vi "PXI_Host_Cluster_40_I8_Read_NewMethod_Benchmark.vi"() -> ()   [LabVIEW 2018]
uses:
  <vilib>/Platform/TimedLoop/XDataNode/timing_clust.ctl
  <vilib>/Platform/TimedLoop/XDataNode/nitl_modes.ctl
  <vilib>/Platform/TimedLoop/XDataNode/wakeup.ctl
  cRIO RT/TypeDefs/Big I8 Cluster.ctl
  acadbf34-ec47-4be6-aee9-0dde4c7960f7.vi
  cRIO RT/FPGA Bitfile Register Operations/Scalar IO Operations/SubVIs/Convert Cluster BLOB to Bool Array.vi
  cRIO RT/FPGA Bitfile Register Operations/Scalar IO Operations/SubVIs/Parse Cluster Configuration.vi
  cRIO RT/FPGA Bitfile Register Operations/Scalar IO Operations/Read Methods/Read Data Register/Instances/Read U8 Array.vi
  acadbf34-ec47-4be6-aee9-0dde4c7960f7.vi/8df46875-ca50-46a7-81d4-ea56393d8c37.vi
  cRIO RT/FPGA Bitfile Register Operations/Scalar IO Operations/SubVIs/Check Cluster Configuration Store.vi
  cRIO RT/FPGA Bitfile Register Operations/Scalar IO Operations/Utilities/Find Register Offset.vi
  cRIO RT/FPGA Bitfile Register Operations/Scalar IO Operations/SubVIs/FXP Raw to DBL.vi
  cRIO RT/FPGA Bitfile Register Operations/Scalar IO Operations/SubVIs/Check Register Data Store.vi
  <userlib>/_OpenG.lib/lvdata/lvdata.llb/Variant to Header Info__ogtk.vi
  <userlib>/_OpenG.lib/lvdata/lvdata.llb/Split Cluster TD__ogtk.vi
  <userlib>/_OpenG.lib/lvdata/lvdata.llb/Cluster to Array of VData__ogtk.vi
  <vilib>/Utility/Data Type/Get Type Information.vi
  <userlib>/_OpenG.lib/lvdata/lvdata.llb/Get Strings from Enum__ogtk.vi
  cRIO RT/FPGA Bitfile Register Operations/Scalar IO Operations/Error Handling/Error 6004.vi
  <vilib>/Utility/Data Type/Get Fixed-Point Information.vi
  cRIO RT/FPGA Bitfile Register Operations/Scalar IO Operations/Error Handling/Error 6001.vi
  cRIO RT/FPGA Bitfile Register Operations/Scalar IO Operations/Error Handling/Error 6000.vi
  cRIO RT/FPGA Bitfile Register Operations/Scalar IO Operations/Error Handling/Error 6002.vi
  cRIO RT/FPGA Bitfile Register Operations/Scalar IO Operations/Error Handling/Error 6003.vi
  <vilib>/FPGAPlugInAG/Dynamic/niLvFpga_Close_Dynamic.vi
  <vilib>/platform/TimedLoop/XDataNode/XDataNode.xnode
  <vilib>/rvi/interface/nirviCloseFPGA/nirviCloseFPGA.xnode
  cRIO RT/FPGA Bitfile Register Operations/Scalar IO Operations/FPGA Register IO.lvlib
  <vilib>/Platform/TimedLoop/XDataNode/XDNodeRunTimeDep.lvlib
panel:
  out "Waveform Graph":dbl[](graph)
  out "Standard Dev":dbl
  out "Execution time (s)":dbl
  out "Maximum(s)":dbl
  out "error out":errorcluster
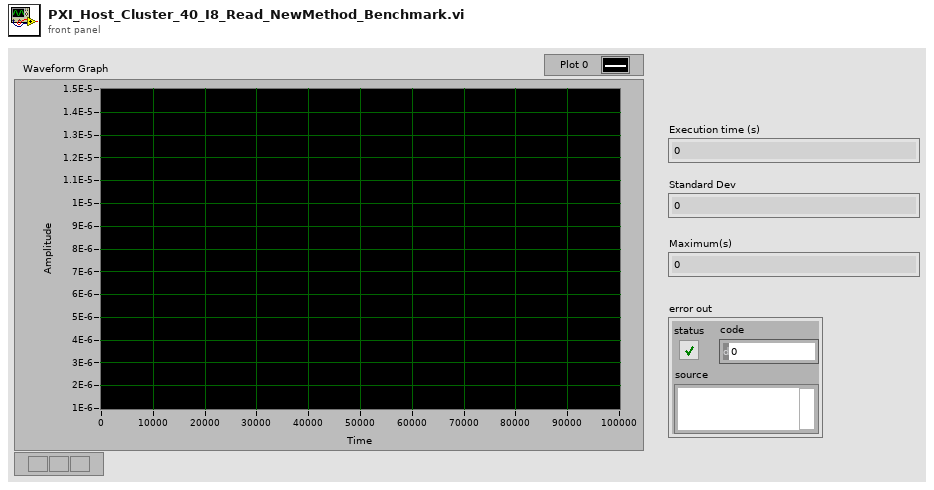
[diagram p1: front panel]
types:
  T1 = typedef "XDNodeRunTimeDep.lvlib/timing_clust.ctl" = cluster{"Expected End [f-1]":u64, "Actual End [f-1]":u64, "Finished Late? [f-1]":bool, "Expected End [i-1]":u64, "Actual End [i-1]":u64, "Finished Late? [i-1]":bool, "Expected Start [i]":u64, "Actual Start [i]":u64, "Expected Start [f]":u64, "Actual Start [f]":u64, "Source Name":string, "Structure Name":string, "Period":i64, "Deadline":i64, "Offset":i64, "Start":i64, "Priority":i32, "Timeout":i32, "Mode":T2, "Wakeup Reason":T3, "Error":errorcluster, "Source Type":string, "Secondary Source Type":string, "Global End Time":u64, "Global Start Time":u64, "Frame Duration":u64, "Iteration Duration":u64, "Assigned CPU":i32, "I/O Scan Engine Mode":u32}
  T2 = typedef "XDNodeRunTimeDep.lvlib/nitl_modes.ctl" = enum32{"No Change", "Process missed periods, maintain original phase", "Discard missed periods, maintain original phase", "Process missed periods, ignore original phase", "Discard missed periods, ignore original phase"}
  T3 = typedef "XDNodeRunTimeDep.lvlib/wakeup.ctl" = enum32{"Normal", "Aborted", "Asynchronous wakeup", "Timing source error", "Timed loop error", "Timeout"}
  T4 = typedef "Big I8 Cluster.ctl" = cluster{"Channel 1":i8, "Channel 2":i8, "Channel 3":i8, "Channel 4":i8, "Channel 5":i8, "Channel 6":i8, "Channel 7":i8, "Channel 8":i8, "Channel 9":i8, "Channel 10":i8, "Channel 11":i8, "Channel 12":i8, "Channel 13":i8, "Channel 14":i8, "Channel 15":i8, "Channel 16":i8, "Channel 17":i8, "Channel 18":i8, "Channel 19":i8, "Channel 20":i8, "Channel 21":i8, "Channel 22":i8, "Channel 23":i8, "Channel 24":i8, "Channel 25":i8, "Channel 26":i8, "Channel 27":i8, "Channel 28":i8, "Channel 29":i8, "Channel 30":i8, "Channel 31":i8, "Channel 32":i8, "Channel 33":i8, "Channel 34":i8, "Channel 35":i8, "Channel 36":i8, "Channel 37":i8, "Channel 38":i8, "Channel 39":i8, "Channel 40":i8}
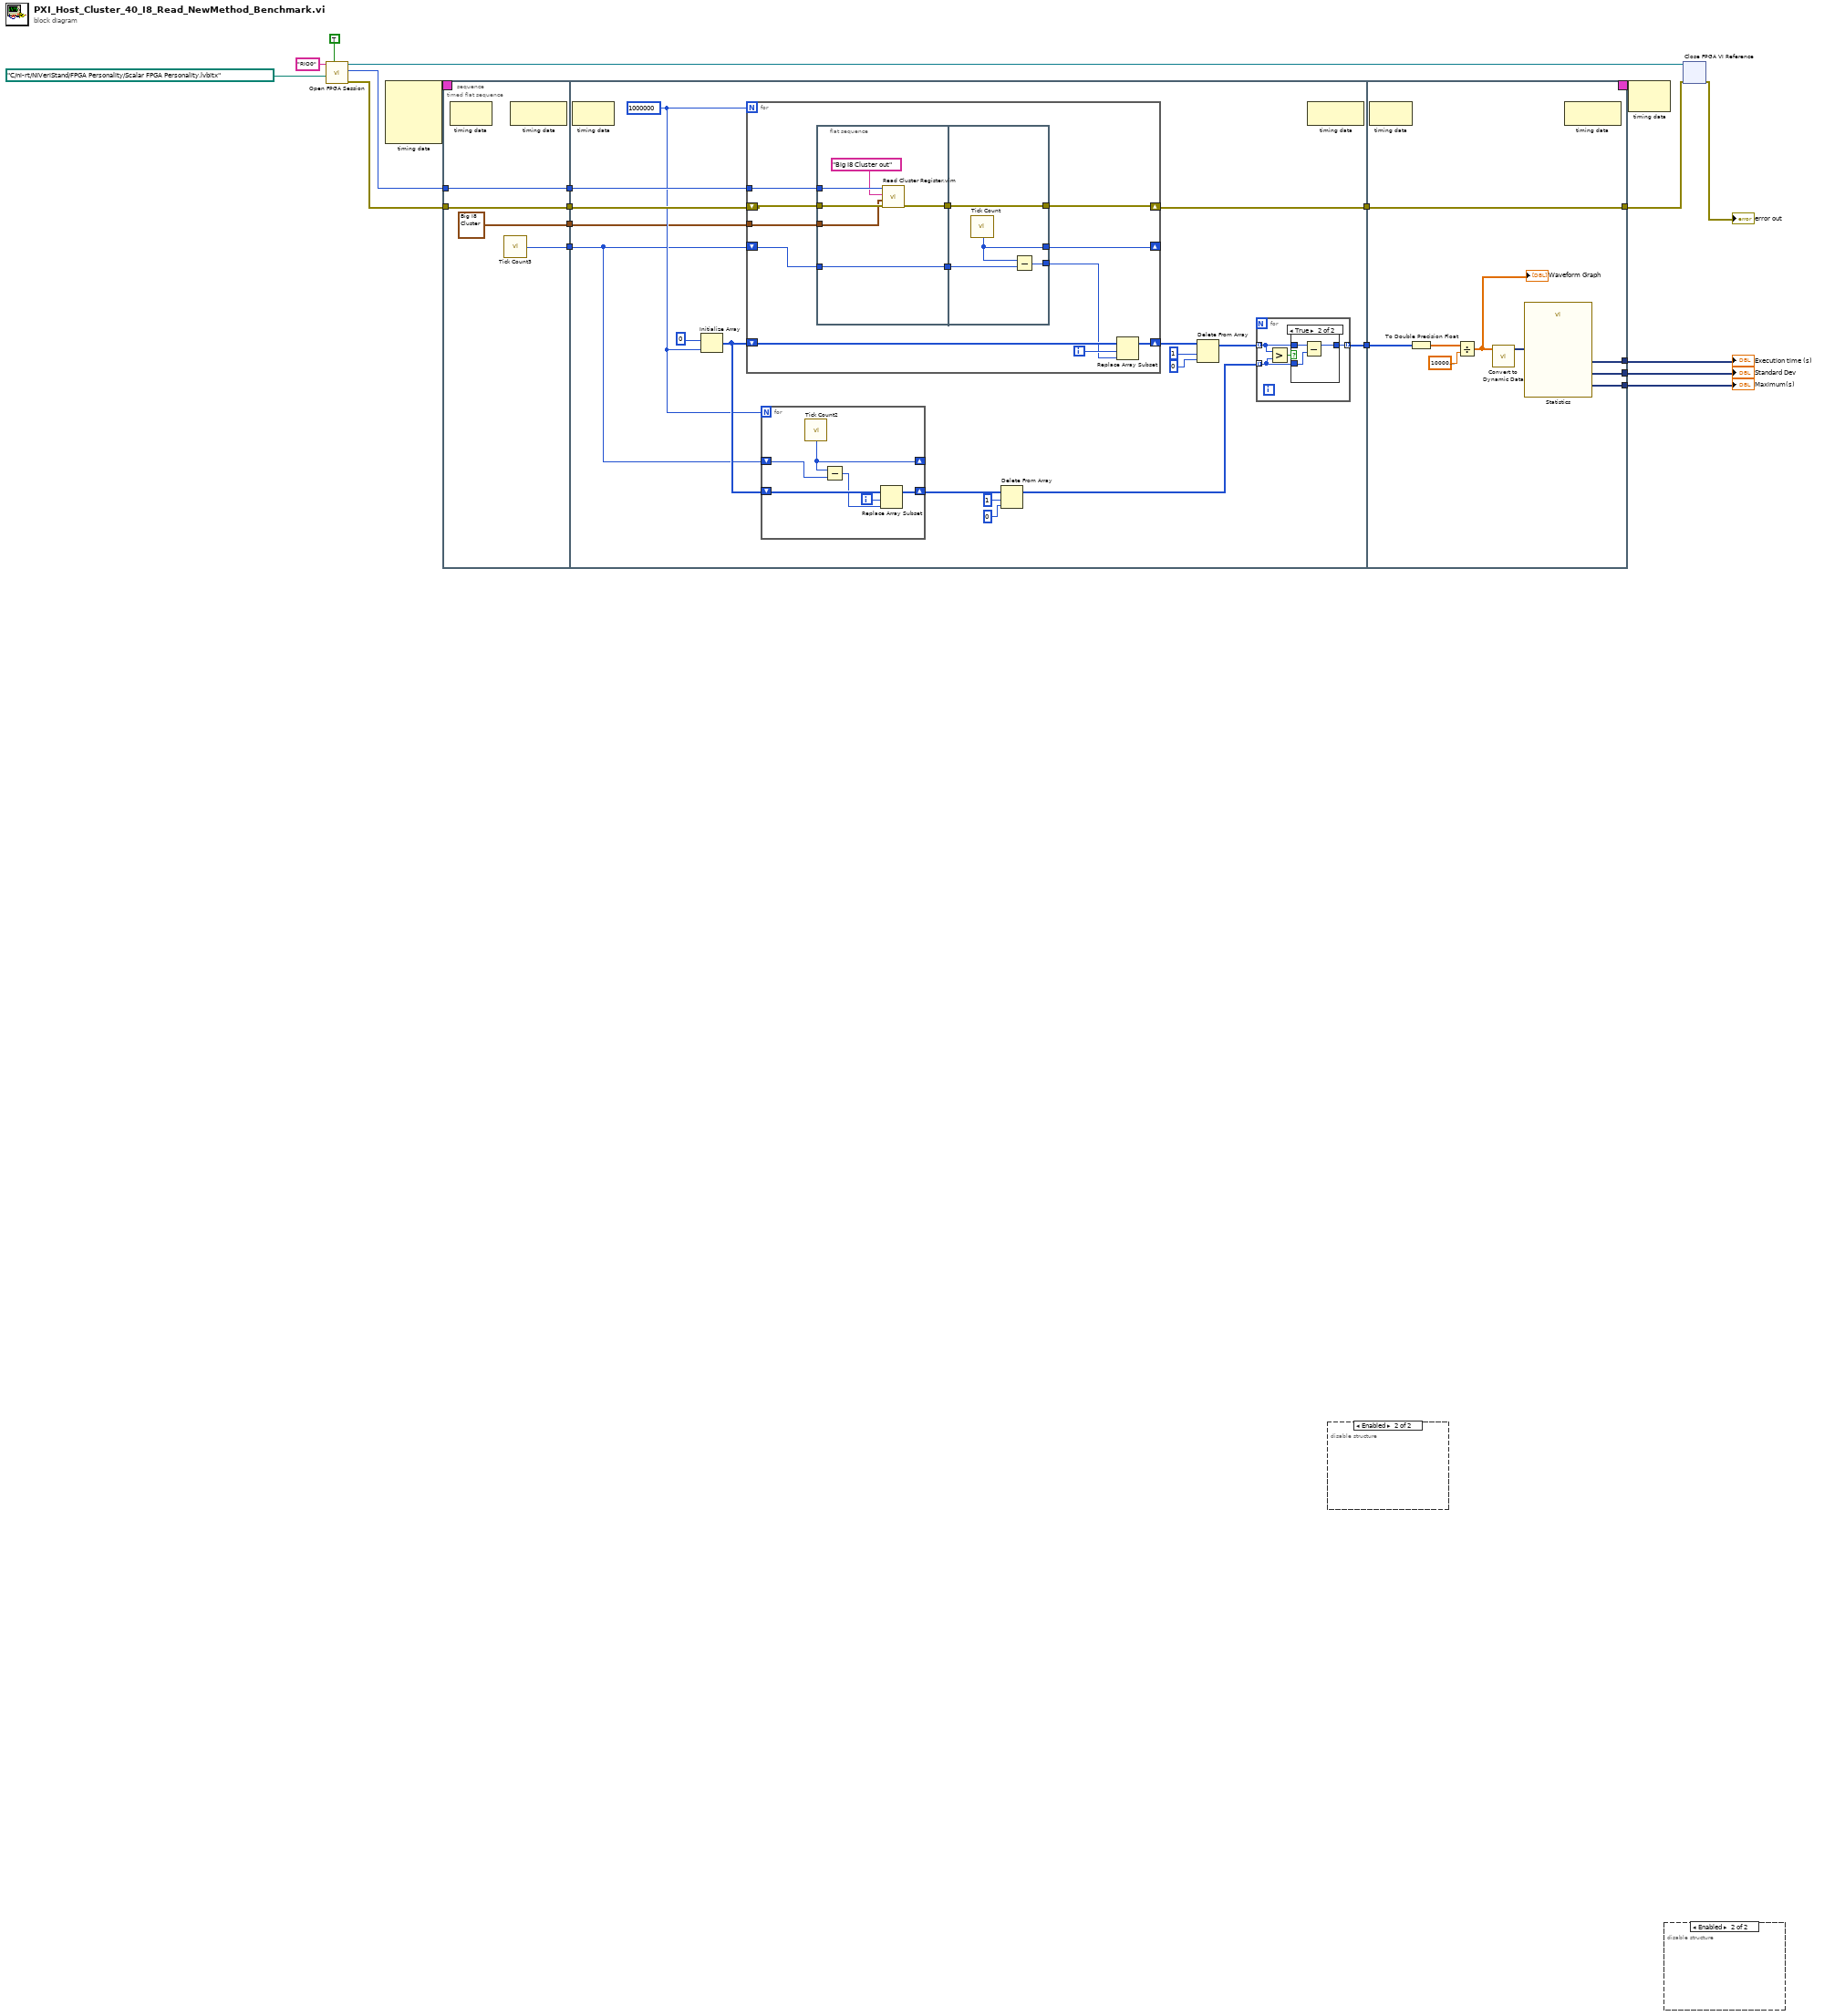
[diagram p0: block diagram]
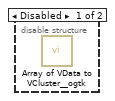
[diagram p3: hidden frame]
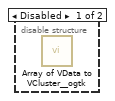
[diagram p4: hidden frame]
diagram:
  n1 = call "Open FPGA Session.vi"("run when loaded (T)"=TRUE, "bitfile path"=path "C:/ni-rt/NIVeriStand/FPGA Personality/Scalar FPGA Personality.lvbitx", "device address"="RIO0") -> ("error out"=w7:errorcluster, "session out"=w11:u32, "bitfile reference out"=w6:refnum<k20>)  [unwired: 6 in]
  n2 = node-c288() -> (w13:T1)  [unwired: 4 in]
  n3 = timed-sequence {
    timing: w13 -> [_]
    timing-out: [_] -> w12
    tunnel: w11 -> [w25]
    tunnel: w7 -> [w24]
    tunnel: [w23] -> w5
    tunnel: [w17] -> w3
    tunnel: [w16] -> w2
    tunnel: [w15] -> w1
    n4 = timed-flat-sequence {
      tunnel: w24 -> [w28]
      tunnel: w25 -> [w29]
      tunnel: [w29] -> w22
      tunnel: [w28] -> w21
      tunnel: [w27] -> w20
      tunnel: [T4 {"Channel 1"=0, "Channel 2"=0, "Channel 3"=0, "Channel 4"=0, "Channel 5"=0, "Channel 6"=0, "Channel 7"=0, "Channel 8"=0, "Channel 9"=0, "Channel 10"=0, "Channel 11"=0, "Channel 12"=0, "Channel 13"=0, "Channel 14"=0, "Channel 15"=0, "Channel 16"=0, "Channel 17"=0, "Channel 18"=0, "Channel 19"=0, "Channel 20"=0, "Channel 21"=0, "Channel 22"=0, "Channel 23"=0, "Channel 24"=0, "Channel 25"=0, "Channel 26"=0, "Channel 27"=0, "Channel 28"=0, "Channel 29"=0, "Channel 30"=0, "Channel 31"=0, "Channel 32"=0, "Channel 33"=0, "Channel 34"=0, "Channel 35"=0, "Channel 36"=0, "Channel 37"=0, "Channel 38"=0, "Channel 39"=0, "Channel 40"=0} ("Big I8 Cluster")] -> w14
      tunnel: w22 -> [w48]
      tunnel: w21 -> [w47]
      tunnel: w20 -> [w33]
      tunnel: [w46] -> w19
      tunnel: [w35] -> w18
      tunnel: w14 -> [w32]
      tunnel: [w95] -> w23
      tunnel: w19 -> [w95]
      tunnel: w18 -> [w91]
      tunnel: [w90] -> w17
      tunnel: [w89] -> w16
      tunnel: [w88] -> w15
      frame #0 {
        n5 = node-c288() -> ()  [unwired: 1 in, 1 out]
        n6 = call "Tick Count3"() -> ("Tick Count(Ticks)"=w27:u32)
        n7 = node-c288() -> ()  [unwired: 1 in, 1 out]
      }
      frame #1 {
        w34 = 1000000
        n8 = node-c288() -> ()  [unwired: 1 in, 1 out]
        n9 = Initialize Array(u32 0 ("Tick Count(uSec)"), w34) -> (w44:u32[])
        n10 = for {
          N: w34 -> [_]
          tunnel: w48 -> [w69]
          shift-right: [w60] -> w46
          shift-left: w47 -> [w68]
          shift-right: [w65] -> w38
          shift-left: w44 -> [w67]
          shift-right: [w62] -> _
          shift-left: w33 -> [w64]
          tunnel: w32 -> [w59]
          i -> [w66]
          n11 = flat-sequence {
            tunnel: [w76] -> w70
            tunnel: w64 -> [w76]
            tunnel: w69 -> [w74]
            tunnel: w68 -> [w75]
            tunnel: [w72] -> w61
            tunnel: w59 -> [w71]
            tunnel: w70 -> [w80]
            tunnel: [w79] -> w63
            tunnel: [w78] -> w62
            tunnel: w61 -> [w77]
            tunnel: [w77] -> w60
            frame #0 {
              n12 = call "Read Cluster Register.vim"("error in (no error)"=w75, "Cluster in (default value)"=w71, "Cluster Name"="Big I8 Cluster out" ("register name"), "session in"=w74) -> ("error out"=w72:errorcluster)  [unwired: 5 in, 2 out]
            }
            frame #1 {
              n13 = call "Tick Count"() -> ("Tick Count(Ticks)"=w78:u32)
              n14 = Subtract(x=w78, y=w80) -> (x-y=w79:u32)
            }
          }
          n15 = Replace Array Subset(array=w67, new element=w63, index=w66) -> (w65:u32[])
        }
        n16 = for {
          N: w34 -> [_]
          shift-right: [w81] -> w41
          shift-left: w44 -> [w84]
          shift-right: [w86] -> _
          shift-left: w33 -> [w85]
          i -> [w82]
          n17 = call "Tick Count2"() -> ("Tick Count(Ticks)"=w86:u32)
          n18 = Subtract(x=w86, y=w85) -> (x-y=w83:u32)
          n19 = Replace Array Subset(array=w84, new element=w83, index=w82) -> (w81:u32[])
        }
        n20 = Delete From Array(array=w41, length=1, index=0) -> (array with subset deleted=w36:u32[])  [unwired: 1 out]
        n21 = Delete From Array(array=w38, length=1, index=0) -> (array with subset deleted=w37:u32[])  [unwired: 1 out]
        n22 = for {
          tunnel: [w54] -> w35 mode=indexing
          tunnel: w37 -> [w53] mode=indexing
          tunnel: w36 -> [w52] mode=indexing
          n23 = Greater?(x=w53, y=w52) -> (0:w51:bool)
          n24 = case shown="True" w51 {
            tunnel: w53 -> [w55 w58]
            tunnel: w52 -> [_ w57]
            tunnel: [w55 w56] -> w54
            frame False {
            }
            frame True {
              n25 = Subtract(x=w58, y=w57) -> (x-y=w56:u32)
            }
          }
        }
        n26 = node-c288() -> ()  [unwired: 1 in, 1 out]
      }
      frame #2 {
        n27 = node-c288() -> ()  [unwired: 1 in, 1 out]
        n28 = To Double Precision Float(number=w91) -> (double precision float=w94:dbl[])
        n29 = Divide(x=w94, y=1000000000.0) -> (x/y=w87:dbl[])
        "Waveform Graph" <- w87
        n30 = call "Convert to Dynamic Data"("Array"=w87) -> ("Dynamic Data Type"=w92:dynamicdata)  [unwired: 3 in]
        n31 = call "Statistics"("Signals"=w92) -> ("Standard Dev"=w89:dynamicdata, "Arithmetic Mean"=w90:dynamicdata, "Maximum"=w88:dynamicdata)  [unwired: 23 in, 1 out]
        n32 = node-c288() -> ()  [unwired: 1 in, 1 out]
      }
    }
  }
  "Maximum(s)" <- w1
  "Execution time (s)" <- w3
  "Standard Dev" <- w2
  n33 = disable-structure shown="Enabled" {
    frame Disabled {
      n34 = call <userlib>:"Array of VData to VCluster__ogtk.vi"() -> ()  [unwired: 10 in, 2 out]
    }
    frame Enabled {
    }
  }
  n35 = node-c288(w12) -> ()  [unwired: 1 out]
  n36 = disable-structure shown="Enabled" {
    frame Disabled {
      n37 = call <userlib>:"Array of VData to VCluster__ogtk.vi"() -> ()  [unwired: 10 in, 2 out]
    }
    frame Enabled {
    }
  }
  n38 = xnode "Close FPGA VI Reference"("FPGA VI Reference In"=w6, "error in"=w5) -> ("error out"=→"error out":errorcluster)
